vi "Add Frame Configuration.vi"(8 "error in (no error)":errorcluster, 11 "Node Ptr":u64 format="%.0x") -> (0 "error out":errorcluster)   [LabVIEW 2021, in "LIN Frame Protection Addon System Explorer.lvlib"]
uses:
  LIN Frame Protection Addon System Explorer.lvlib
  <vilib>/NI VeriStand/Custom Device API/Custom Device Channel.ctl
  <vilib>/NI VeriStand/Custom Device API/Custom Device Channel Type.ctl
  Shared/SubVIs/GUID Lookup.vi
  <vilib>/NI VeriStand/Custom Device API/Custom Device API.lvlib
  Shared/LIN Frame Protection Addon Shared.lvlib
panel:
  in  "Tag":string
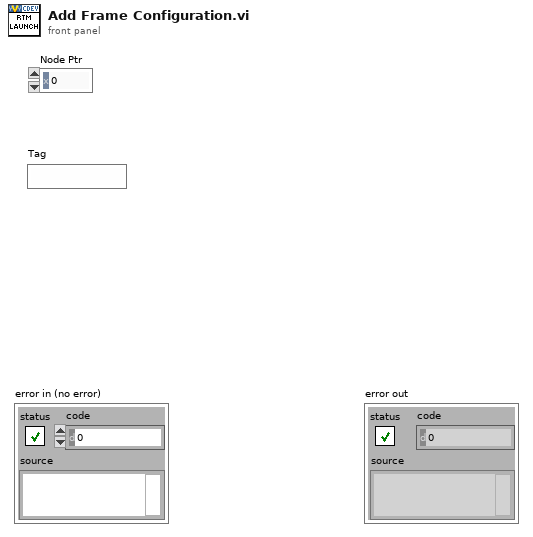
[diagram p1: front panel]
types:
  T1 = typedef "Custom Device API.lvlib/Custom Device Item Ref.ctl" = u64
  T2 = typedef "Custom Device API.lvlib/Custom Device Channel.ctl" = cluster{"Type":T3, "Units":string, "Default Value":dbl, "Faultable":bool, "Scalable":bool}
  T3 = typedef "Custom Device API.lvlib/Custom Device Channel Type.ctl" = enum16{"Input", "Output"}
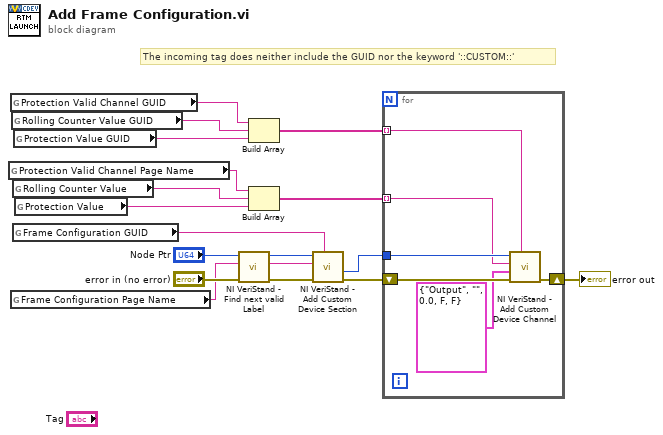
[diagram p0: block diagram]
diagram:
  # "The incoming tag does neither include the GUID nor the keyword '::CUSTOM::'"
  n1 = global read "GUID Lookup.vi" "Protection Valid Channel Page Name"() -> (w1:string)
  n2 = global read "GUID Lookup.vi" "Protection Valid Channel GUID"() -> (w2:string)
  n3 = global read "GUID Lookup.vi" "Frame Configuration Page Name"() -> (w14:string)
  n4 = global read "GUID Lookup.vi" "Rolling Counter Value GUID"() -> (w5:string)
  n5 = global read "GUID Lookup.vi" "Rolling Counter Value"() -> (w7:string)
  n6 = global read "GUID Lookup.vi" "Frame Configuration GUID"() -> (w12:string)
  n7 = global read "GUID Lookup.vi" "Protection Value GUID"() -> (w4:string)
  n8 = global read "GUID Lookup.vi" "Protection Value"() -> (w8:string)
  n9 = call <vilib>:"NI VeriStand - Find next valid Label.vi"("error in (no error)"="error in (no error)", "Label"=w14, "Item Ref in"="Node Ptr") -> ("error out"=w16:errorcluster, "Label out"=w13:string, "Item Ref out"=w18:T1)  [unwired: 4 in, 2 out]
  n10 = Build Array(w2, w5, w4) -> (w3:string[])
  n11 = Build Array(w1, w7, w8) -> (w6:string[])
  n12 = call <vilib>:"NI VeriStand - Add Custom Device Section.vi"("GUID (Default Section)"=w12, "error in (no error)"=w16, "Section Name"=w13, "Parent Ref in"=w18) -> ("error out"=w11:errorcluster, "Section Ptr"=w9:T1)  [unwired: 4 in, 2 out]
  n13 = for {
    shift-right: [w23] -> w10
    shift-left: w11 -> [w24]
    tunnel: w9 -> [w22]
    tunnel: w6 -> [w20] mode=indexing
    tunnel: w3 -> [w19] mode=indexing
    n14 = call <vilib>:"NI VeriStand - Add Custom Device Channel.vi"("GUID (Default Channel)"=w19, "error in (no error)"=w24, "Channel"=T2 {"Type"=enum."Output", "Units"="", "Default Value"=0.0, "Faultable"=FALSE, "Scalable"=FALSE}, "Channel Name"=w20, "Parent Ref in"=w22) -> ("error out"=w23:errorcluster)  [unwired: 3 in, 3 out]
  }
  "error out" <- w10
